vi "Actor Core.vi"(8 "error in":errorcluster, 11 "Field Drawer in":refnum<class "Field Drawer.lvclass">) -> (0 "error out":errorcluster, 3 "Actor out":refnum<class "Actor.lvclass">)   [LabVIEW 2022 SP3, in "Vision.lvlib" / "Field Drawer.lvlib" / "Field Drawer.lvclass"]
doc: "(<B>Filename</B>: Actor Framework.lvlib:Actor.lvclass:Actor Core.vi)\n\nReceives messages to the actor, reacts to them, and initiates any error handling that may shut the actor down.\n\nDescendant classes may override this VI to append parallel tasks for the actor to complete while it handles messages. Overrides use the Call Parent Class Method node."
uses:
  Field Drawer.lvclass
  C:/Program Files (x86)/National Instruments/LabVIEW 2022/vi.lib/ActorFramework/Actor/Actor.lvclass
  <vilib>/ActorFramework/Actor/Actor.lvclass
  Old vision/Controls/Field Size.ctl
  Field Drawer.lvclass/Field Drawer.ctl
  <vilib>/ActorFramework/Actor/Actor.lvclass/Actor.ctl
  <vilib>/ActorFramework/Message Enqueuer/Message Enqueuer.lvclass/Message Enqueuer.ctl
  Messages/Draw Field_Msg/Draw Field_Msg.lvclass/Draw Field_Msg.ctl
  Vision/Vision Messages/Update Drawing Msg/Update Drawing Msg.lvclass/Update Drawing Msg.ctl
  <vilib>/ActorFramework/Message Enqueuer/Init from Existing Queue.vi
  <vilib>/ActorFramework/Message Enqueuer/Enqueue.vi
  Messages/Draw Field_Msg/Draw Field_Msg.lvclass
  C:/Program Files (x86)/National Instruments/LabVIEW 2022/vi.lib/ActorFramework/Message/Message.lvclass
  Vision/Vision Messages/Update Drawing Msg/Update Drawing Msg.lvclass
  <vilib>/ActorFramework/Message Priority Queue/Priority Enqueue.vi
  <vilib>/MGI/Monitored Actor/Monitored Actor/Monitored Actor/Monitored Actor.lvclass
  <vilib>/ActorFramework/Message Enqueuer/Message Enqueuer.lvclass
  C:/Program Files (x86)/National Instruments/LabVIEW 2022/vi.lib/MGI/Monitored Actor/Monitored Actor/Monitored Actor/Monitored Actor.lvclass
  C:/Users/ebert/Documents/codes/SSL/repo/Phoenix Reborn/Field Drawer/Field Drawer/Field Drawer.lvclass
panel:
  in  "Field Size":T1
  in  "Scale":dbl=0.09
  out "Field Drawing":picture
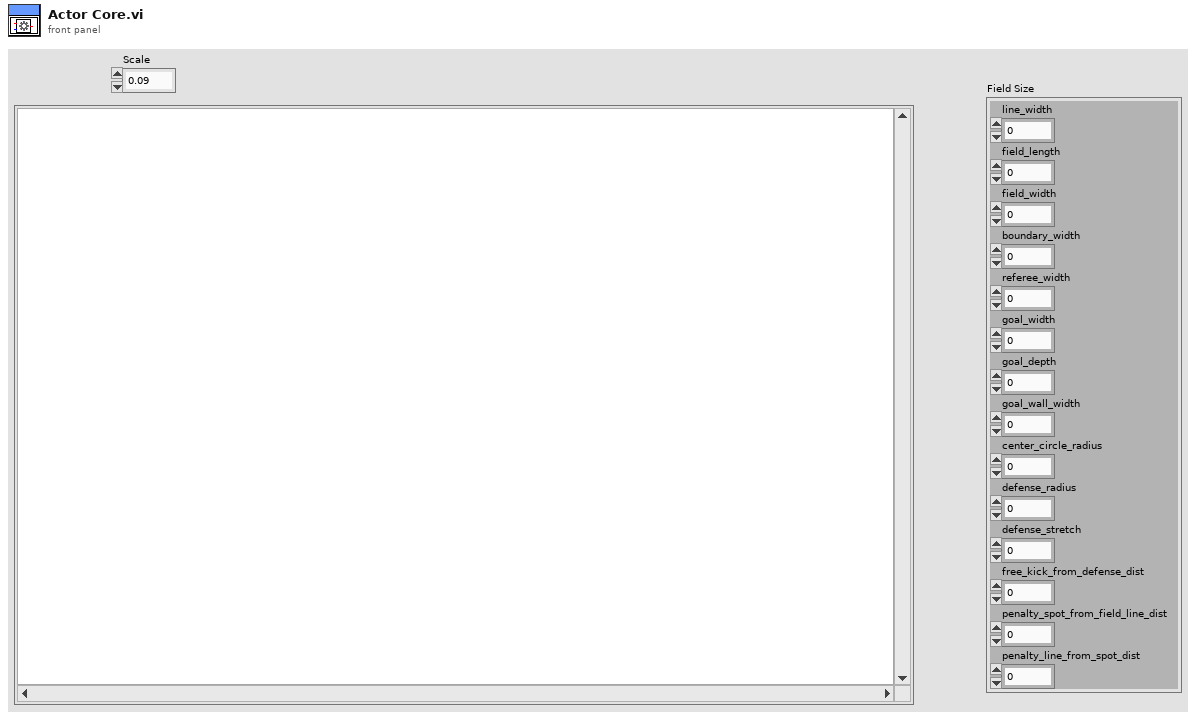
[diagram p1: front panel]
types:
  T1 = typedef "Field Size.ctl" = cluster{"line_width":u32, "field_length":u32, "field_width":u32, "boundary_width":u32, "referee_width":u32, "goal_width":u32, "goal_depth":u32, "goal_wall_width":u32, "center_circle_radius":u32, "defense_radius":u32, "defense_stretch":u32, "free_kick_from_defense_dist":u32, "penalty_spot_from_field_line_dist":u32, "penalty_line_from_spot_dist":u32}
  T2 = cluster{"Stop":refnum<user-event>, "Halt":refnum<user-event>, "Start":refnum<user-event>}
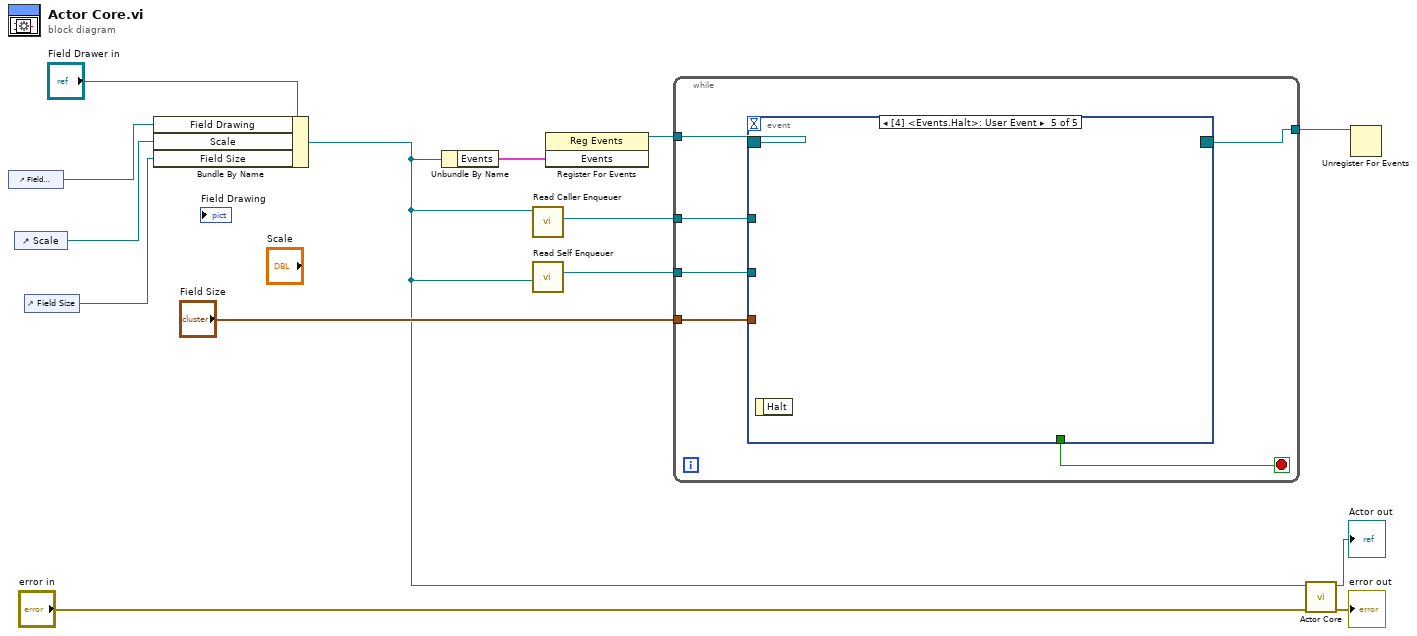
[diagram p0: block diagram]
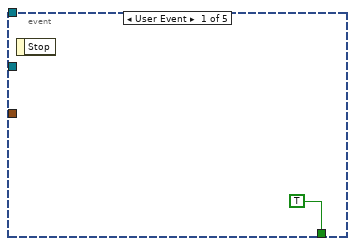
[diagram p2: hidden frame]
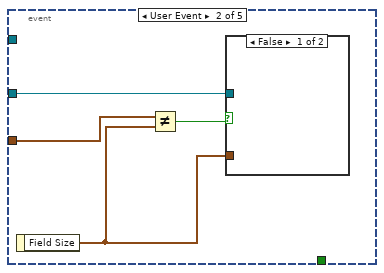
[diagram p3: hidden frame]
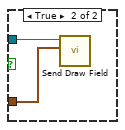
[diagram p4: hidden frame]
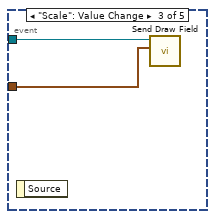
[diagram p5: hidden frame]
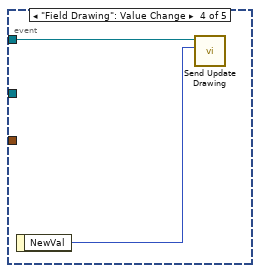
[diagram p6: hidden frame]
diagram:
  n1 = control-ref of="Field Drawing"() -> (w6:refnum<vi>)
  n2 = control-ref of="Scale"() -> (w5:refnum<vi>)
  n3 = control-ref of="Field Size"() -> (w4:refnum<vi>)
  n4 = Bundle By Name(cluster="Field Drawer in", "Field Drawing"=w6, "Scale"=w5, "Field Size"=w4) -> (w2:refnum<class "Field Drawer.lvclass">)
  n5 = Unbundle By Name(w2) -> ("Events"=w11:T2)
  n6 = call <vilib>:"Read Caller Enqueuer.vi"("Actor"=w2) -> ("Caller Enqueuer"=w1:refnum<class "Message Enqueuer.lvclass">)  [unwired: 10 in]
  n7 = call <vilib>:"Read Self Enqueuer.vi"("Actor"=w2) -> ("Self Enqueuer"=w8:refnum<class "Message Enqueuer.lvclass">)  [unwired: 10 in]
  n8 = register-events(w11) -> (reference out=w10:refnum<event-registration>)  [unwired: 2 in, 1 out]
  n9 = while {
    tunnel: w10 -> [w20]
    tunnel: [w19] -> w9
    tunnel: w8 -> [w17]
    tunnel: "Field Size" -> [w16]
    tunnel: w1 -> [w15]
    stop <- w18 stop-if-true
    n10 = event shown="[4] <Events.Halt>: User Event" {
      selector: w20 -> [_ _ _ _ _]
      dyn-events: [_ _ _ _ _] -> w19
      timeout: _ -> [_ _ _ _ _]
      tunnel: [TRUE _ _ _ _] -> w18
      tunnel: w17 -> [_ w25 w29 _ _]
      tunnel: w16 -> [_ w22 w28 _ _]
      tunnel: w15 -> [_ _ _ w31 _]
      event User Event {
        n11 = event-data() -> ()  [unwired: 1 in, 1 out]
      }
      event User Event {
        n12 = event-data() -> ("Field Size"=w23:T1)  [unwired: 1 in]
        n13 = Not Equal?(x=w22, y=w23) -> (x != y?=w24:bool)
        n14 = case shown="False" w24 {
          tunnel: w23 -> [_ w27]
          tunnel: w25 -> [_ w26]
          frame False {
          }
          frame True {
            n15 = call "Send Draw Field.vi"("Field Size 2"=w27, "Message Enqueuer"=w26) -> ()  [unwired: 8 in, 2 out]
          }
        }
      }
      event "Scale": Value Change {
        n16 = event-data() -> ()  [unwired: 1 in, 1 out]
        n17 = call "Send Draw Field.vi"("Field Size 2"=w28, "Message Enqueuer"=w29) -> ()  [unwired: 8 in, 2 out]
      }
      event "Field Drawing": Value Change {
        n18 = event-data() -> ("NewVal"=w30:picture)  [unwired: 1 in]
        n19 = call "Send Update Drawing.vi"("Field Drawing"=w30, "Message Enqueuer"=w31) -> ()  [unwired: 8 in, 2 out]
      }
      event User Event {
        n20 = event-data() -> ()  [unwired: 1 in, 1 out]
      }
    }
  }
  n21 = call-parent "Actor Core.vi"("error in"="error in", "Actor in"=w2) -> ("error out"=→"error out":errorcluster, "Actor out"=→"Actor out":refnum<class "Actor.lvclass">)  [unwired: 8 in]
  n22 = Unregister For Events(event registration refnum=w9) -> ()  [unwired: 1 in, 1 out]
